vi "REPORT_OPRTN_prepare_header_for_csv.vi"(11 "REPORT_OPRTN_all_info":T1) -> (3 "report_header":string[][](array[string]))   [LabVIEW 2019]
uses:
  typedef/REPORT_OPRTN_all_info.ctl
  DATES/typedef/REPORT_DATES_statuses.ctl
  _misc/AULocalize/SubVIs/Get Localized Phrase Compact Interface 1D.vi
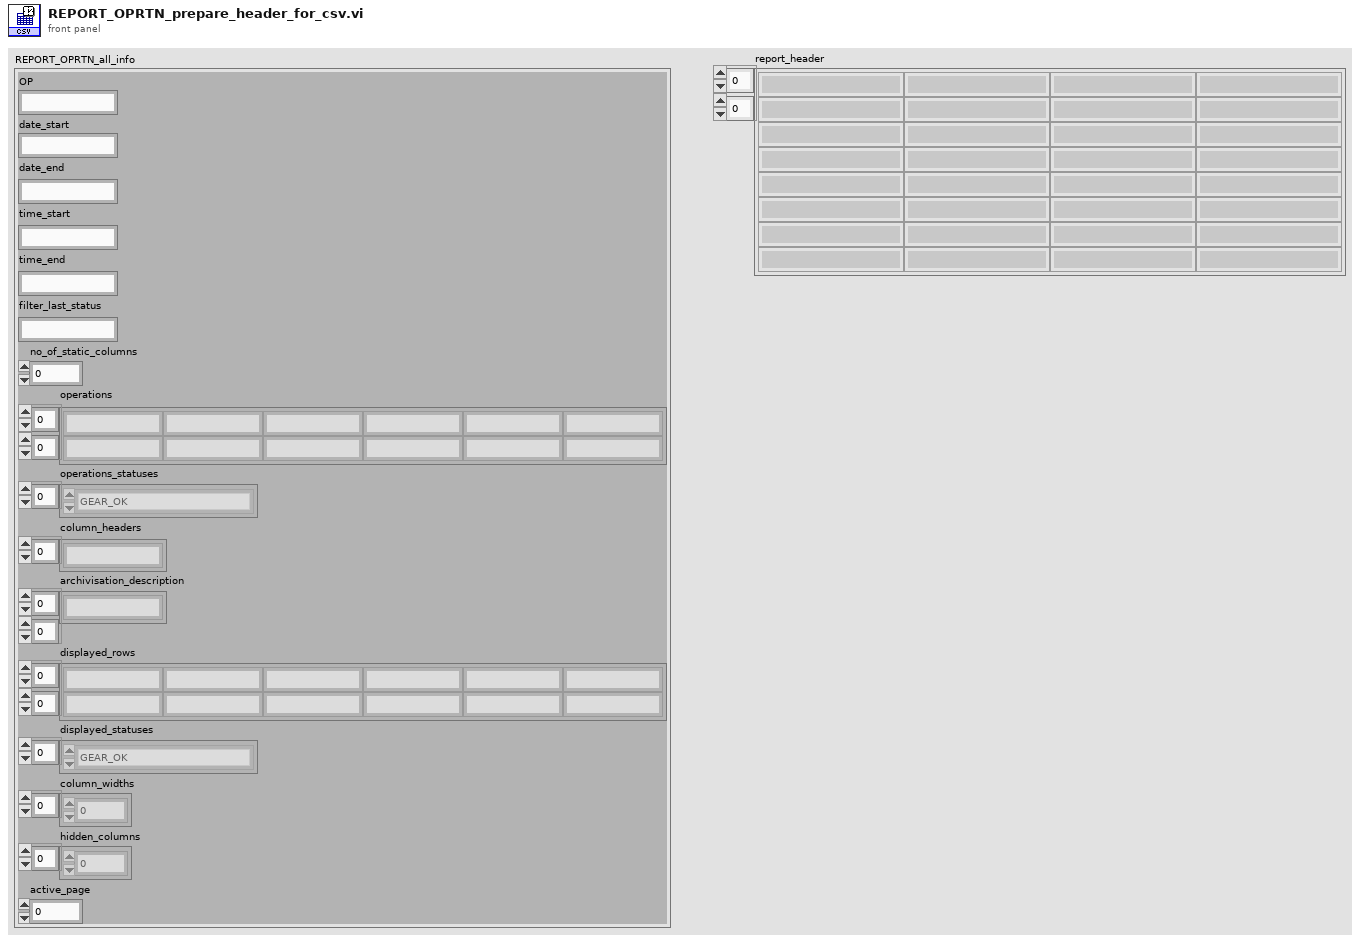
[diagram p1: front panel]
types:
  T1 = typedef "REPORT_OPRTN_all_info.ctl" = cluster{"OP":string, "date_start":string, "date_end":string, "time_start":string, "time_end":string, "filter_last_status":string, "no_of_static_columns":i32, "operations":string[][], "operations_statuses":T2[], "column_headers":string[], "archivisation_description":string[][], "displayed_rows":string[][], "displayed_statuses":T2[], "column_widths":i16[], "hidden_columns":i32[], "active_page":i32}
  T2 = typedef "REPORT_DATES_statuses.ctl" = enum16{"GEAR_OK", "GEAR_NOK", "GEAR_interrupted", "GEAR_in_operation", "GEAR_unexpected"}
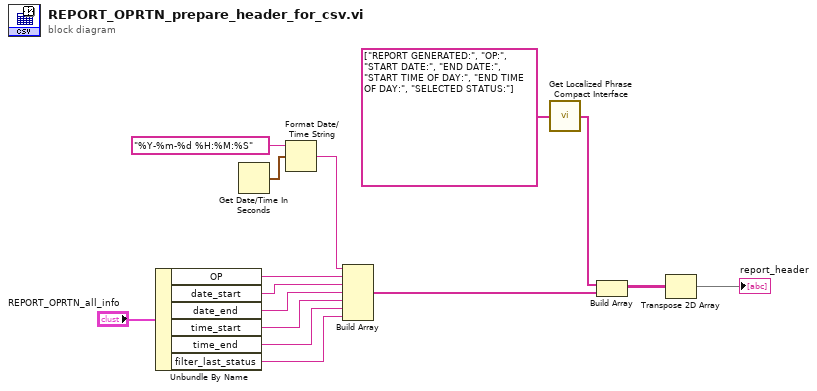
[diagram p0: block diagram]
diagram:
  n1 = Unbundle By Name("REPORT_OPRTN_all_info") -> ("OP"=w9:string, "date_start"=w8:string, "date_end"=w7:string, "time_start"=w4:string, "time_end"=w3:string, "filter_last_status"=w2:string)
  n2 = Get Date/Time In Seconds() -> (seconds since 1Jan1904=w14:timestamp)
  n3 = Format Date/Time String(time format string (%c)="%Y-%m-%d %H:%M:%S", seconds (now)=w14) -> (date/time string=w6:string)  [unwired: 1 in]
  n4 = Build Array(w6, w9, w8, w7, w4, w3, w2) -> (w10:string[])
  n5 = call-poly "Get Localized Phrase Compact Interface.vi"("Key"=string[] ["REPORT GENERATED:", "OP:", "START DATE:", "END DATE:", "START TIME OF DAY:", "END TIME OF DAY:", "SELECTED STATUS:"]) -> ("Translated Phrase"=w1:string[])
  n6 = Build Array(w1, w10) -> (w13:string[][])
  n7 = Transpose 2D Array(2D array=w13) -> (transposed array=→"report_header":string[][])
